vi "Device Launcher - Engine.vi"() -> ()   [LabVIEW 2016]
uses:
  Device Launcher Controls/Device Information.ctl
panel:
  in  "Quit":bool
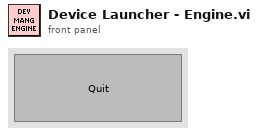
[diagram p1: front panel]
types:
  T1 = typedef "Device Information.ctl" = cluster{"Notifier Name":string, "Device Ports/IDs/Channels":string[], "Device Engine Path":path}
  T2 = enum32{"Invalid", "Standard", "Closed", "Hidden", "Minimized", "Maximized"}
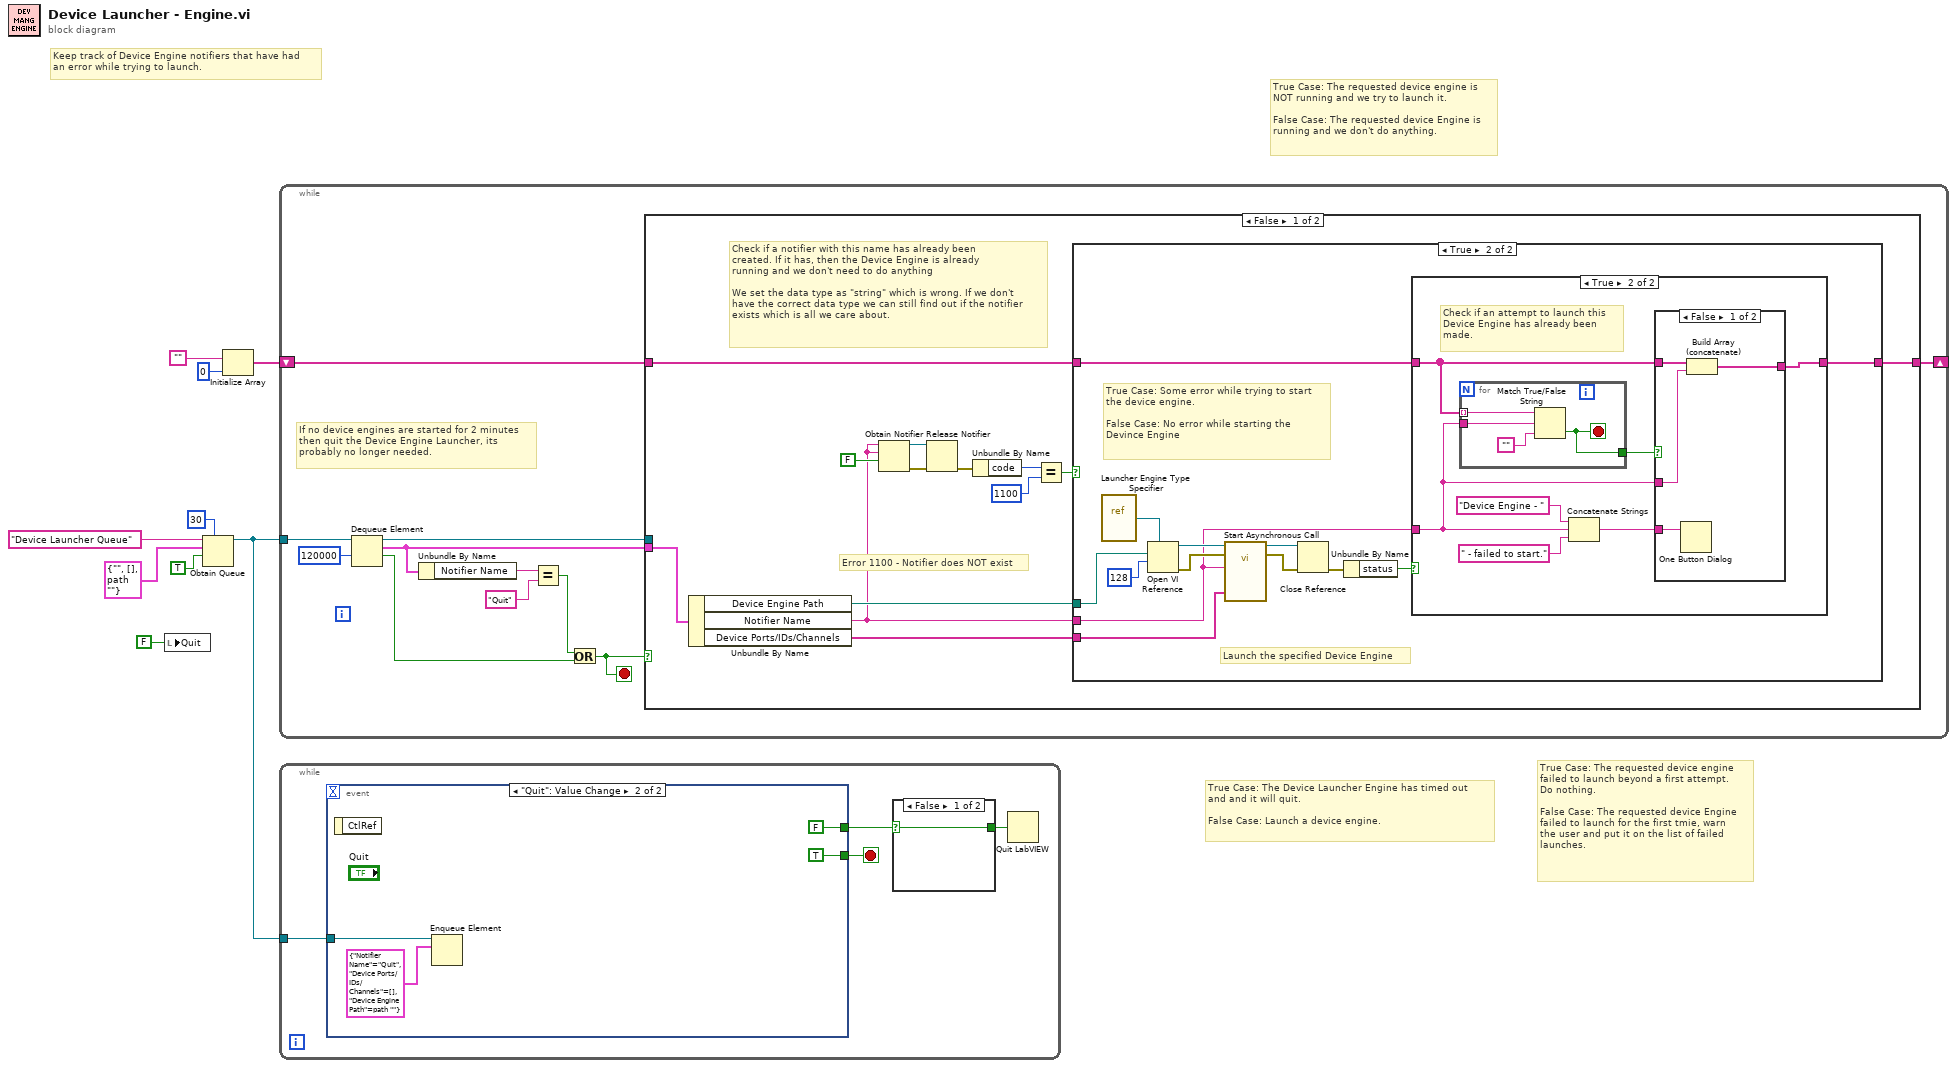
[diagram p0: block diagram]
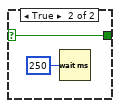
[diagram p2: hidden frame]
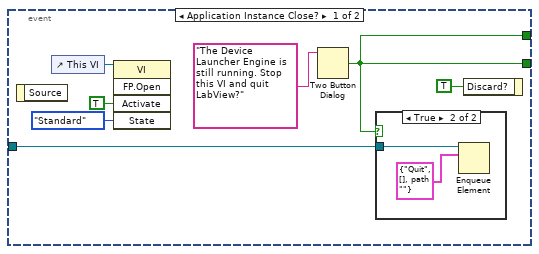
[diagram p3: hidden frame]
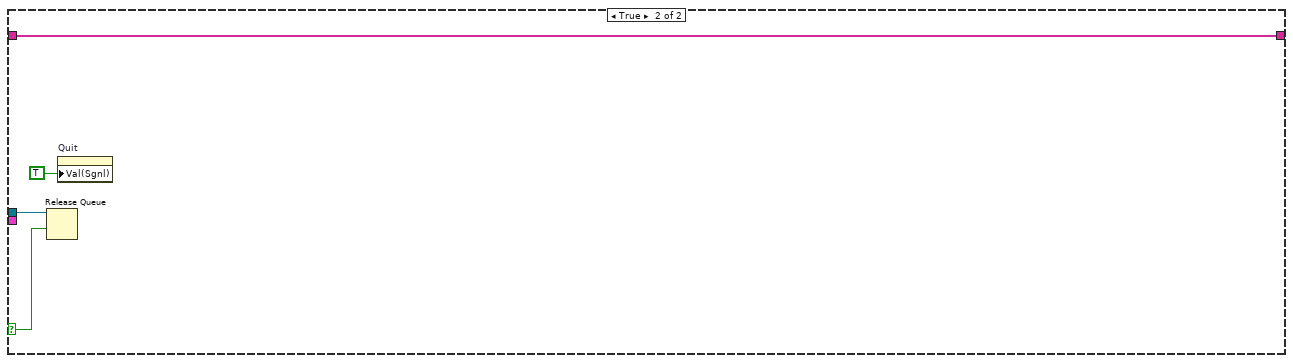
[diagram p8: hidden frame]
diagram:
  # "True Case: The Device Launcher Engine has timed out\nand and it will quit.\n\nFalse Case: Launch a device engine."
  # "True Case: The requested device engine\nfailed to launch beyond a first attempt.\nDo nothing.\n\nFalse Case: The requested device Engine\nfailed to launch for the first tmie, warn\nthe user and put it on the list of failed\nlaunches."
  # "True Case: The requested device engine is\nNOT running and we try to launch it.\n\nFalse Case: The requested device Engine is\nrunning and we don't do anything."
  # "Keep track of Device Engine notifiers that have had\nan error while trying to launch."
  n1 = local write "Quit"(FALSE ("Quit")) -> ()
  n2 = Obtain Queue(max queue size (-1, unlimited)=30, name (unnamed)="Device Launcher Queue", element data type=T1 {"Notifier Name"="", "Device Ports/IDs/Channels"=[], "Device Engine Path"=path ""} ("Device Information"), create if not found? (T)=TRUE) -> (queue out=w2:refnum<queue>)  [unwired: 1 in, 2 out]
  n3 = Initialize Array("", 0 ("dimension size")) -> (w3:string[])
  n4 = while {
    tunnel: w2 -> [w20]
    shift-right: [w18] -> _
    shift-left: w3 -> [w19]
    stop <- w11 stop-if-true
    # "If no device engines are started for 2 minutes\nthen quit the Device Engine Launcher, its\nprobably no longer needed."
    n5 = Dequeue Element(queue=w20, timeout in ms (-1)=120000) -> (queue out=w16:refnum<queue>, element=w15:T1, timed out?=w10:bool)  [unwired: 1 in, 1 out]
    n6 = Unbundle By Name(w15) -> ("Notifier Name"=w14:string)
    n7 = Equal?(x=w14, y="Quit") -> (x = y?=w12:bool)
    n8 = Or(x=w12, y=w10) -> (x .or. y?=w11:bool)
    n9 = case shown="False" w11 {
      selector: w11 -> [_ w66]
      tunnel: w15 -> [w33 _]
      tunnel: w19 -> [w26 w68]
      tunnel: [w25 w68] -> w18
      tunnel: w16 -> [_ w67]
      frame False {
        # "Check if a notifier with this name has already been\ncreated. If it has, then the Device Engine is already\nrunning and we don't need to do anything\n\nWe set the data type as \"string\" which is wrong. If we don't\nhave the correct data type we can still find out if the notifier\nexists which is all we care about."
        # "Error 1100 - Notifier does NOT exist"
        n10 = Unbundle By Name(w33) -> ("Device Engine Path"=w28:path, "Notifier Name"=w27:string, "Device Ports/IDs/Channels"=w29:string[])
        n11 = Obtain Notifier(name (unnamed)=w27, notification data type=w27, create if not found? (T)=FALSE) -> (notifier out=w23:refnum<notifier>, error out=w22:errorcluster)  [unwired: 1 in, 1 out]
        n12 = Release Notifier(notifier=w23, error in (no error)=w22) -> (error out=w21:errorcluster)  [unwired: 1 in, 2 out]
        n13 = Unbundle By Name(w21) -> ("code"=w32:i32)
        n14 = Equal?(x=w32, y=1100) -> (x = y?=w24:bool)
        n15 = case shown="True" w24 {
          tunnel: w27 -> [_ w37]
          tunnel: w29 -> [_ w40]
          tunnel: w28 -> [_ w39]
          tunnel: w26 -> [w34 w36]
          tunnel: [w34 w35] -> w25
          frame False {
          }
          frame True {
            # "Launch the specified Device Engine"
            # "True Case: Some error while trying to start\nthe device engine.\n\nFalse Case: No error while starting the\nDevince Engine"
            n16 = vi-ref "Launcher Engine Type Specifier.vi"() -> (w42:refnum<vi>)
            n17 = Open VI Reference(type specifier VI Refnum (for type only)=w42, vi path=w39, options=128) -> (vi reference=w43:refnum<vi>, error out=w45:errorcluster)  [unwired: 3 in]
            n18 = call-by-ref "Start Asynchronous Call"(reference=w43, error in=w45, "Unique Notifier Name"=w37, "DIO Lines"=w40) -> (reference out=w44:refnum<vi>, error out=w46:errorcluster)  [unwired: 14 in]
            n19 = Close Reference(reference=w44, error in (no error)=w46) -> (error out=w47:errorcluster)
            n20 = Unbundle By Name(w47) -> ("status"=w38:bool)
            n21 = case shown="True" w38 {
              tunnel: w37 -> [_ w52]
              tunnel: w36 -> [w48 w51]
              tunnel: [w48 w49] -> w35
              frame False {
              }
              frame True {
                # "Check if an attempt to launch this\nDevice Engine has already been\nmade."
                n22 = for {
                  tunnel: w51 -> [w64] mode=indexing
                  tunnel: w52 -> [w61]
                  tunnel: [w62] -> w53
                  stop <- w62 stop-if-true
                  n23 = Match True/False String(2:"", 3:w61, 4:w64) -> (0:w62:bool)  [unwired: 1 out]
                }
                n24 = Concatenate Strings("Device Engine - " ("name (unnamed)"), w52, " - failed to start." ("name (unnamed)")) -> (w50:string)
                n25 = case shown="False" w53 {
                  tunnel: w52 -> [w58 _]
                  tunnel: w51 -> [w59 w60]
                  tunnel: [w57 w60] -> w49
                  tunnel: w50 -> [w56 _]
                  frame False {
                    n26 = One Button Dialog(message=w56) -> ()  [unwired: 1 in, 1 out]
                    n27 = Build Array (concatenate)(w59, w58) -> (w57:string[])
                  }
                  frame True {
                  }
                }
              }
            }
          }
        }
      }
      frame True {
        n28 = Release Queue(queue=w67, force destroy? (F)=w66) -> ()  [unwired: 1 in, 3 out]
        n29 = property on="Quit" class="Bool (strict)"("Val(Sgnl)"=TRUE) -> ()  [unwired: 2 in, 2 out]
      }
    }
  }
  n30 = while {
    tunnel: w2 -> [w71]
    stop <- w72 stop-if-true
    n31 = event shown="[1] \"Quit\": Value Change" {
      selector: _ -> [_ _]
      dyn-events: _ -> [_ _]
      timeout: _ -> [_ _]
      tunnel: [w77 TRUE ("T button?")] -> w72
      tunnel: [w77 FALSE ("T button?")] -> w70
      tunnel: w71 -> [w76 w86]
      event Application Instance Close? {
        n32 = event-data() -> ()  [unwired: 1 in, 1 out]
        n33 = control-ref of="This VI"() -> (w81:refnum<vi>)
        n34 = invoke class="VI" method="FP.Open"(reference=w81, "Activate"=TRUE ("Activate?"), "State"=T2."Standard") -> ()  [unwired: 2 in, 5 out]
        n35 = Two Button Dialog(message="The Device Launcher Engine is still running. Stop this VI and quit LabView?") -> (T button?=w77:bool)  [unwired: 2 in]
        n36 = case shown="True" w77 {
          tunnel: w76 -> [_ w83]
          frame False {
          }
          frame True {
            n37 = Enqueue Element(queue=w83, element=T1 {"Notifier Name"="Quit", "Device Ports/IDs/Channels"=[], "Device Engine Path"=path ""} ("Quit Constant")) -> ()  [unwired: 2 in, 3 out]
          }
        }
        n38 = event-data("Discard?"=TRUE) -> ()  [unwired: 1 in, 1 out]
      }
      event "Quit": Value Change {
        n39 = event-data() -> ()  [unwired: 1 in, 1 out]
        n40 = Enqueue Element(queue=w86, element=T1 {"Notifier Name"="Quit", "Device Ports/IDs/Channels"=[], "Device Engine Path"=path ""} ("Device Information")) -> ()  [unwired: 2 in, 3 out]
      }
    }
    n41 = case shown="False" w70 {
      selector: w70 -> [w73 w75]
      tunnel: [w73 w75] -> w69
      frame False {
      }
      frame True {
        n42 = Wait (ms)(milliseconds to wait=u32 250) -> ()  [unwired: 1 out]
      }
    }
    n43 = Quit LabVIEW(quit? (T)=w69) -> ()
  }
